vi "Dead Pixel Detection.vi"(0 "image in":refnum<class "MSC Image.lvclass">, 5 "error in (no error)":errorcluster) -> (14 "image out":refnum<class "MSC Image.lvclass">, 15 "mask image out":refnum<class "MSC Image.lvclass">, 19 "error out":errorcluster)   [LabVIEW 2016, in "MSC Image.lvclass"]
doc: "Detects dead pixels through a simple thesholding operation. Use an image with maximum illumination.\n\nYou can use the mask image of the detected pixels with Inpaint to restore the fragments."
uses:
  MSC Image.lvclass
  controls/Image Type.ctl
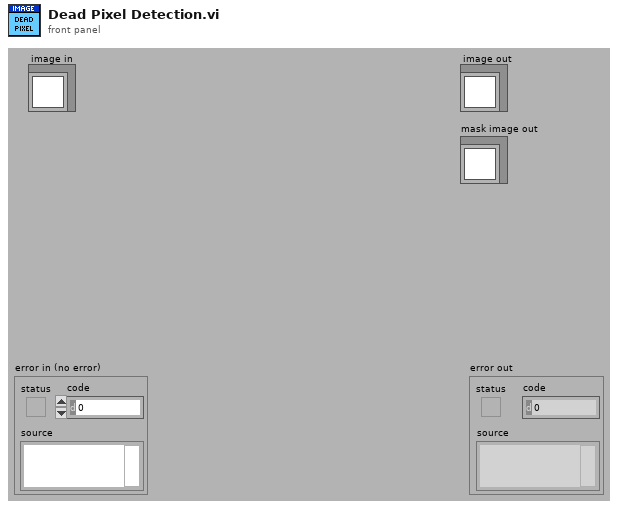
[diagram p1: front panel]
types:
  T1 = typedef "MSC Image.lvclass/Image Type.ctl" = i32
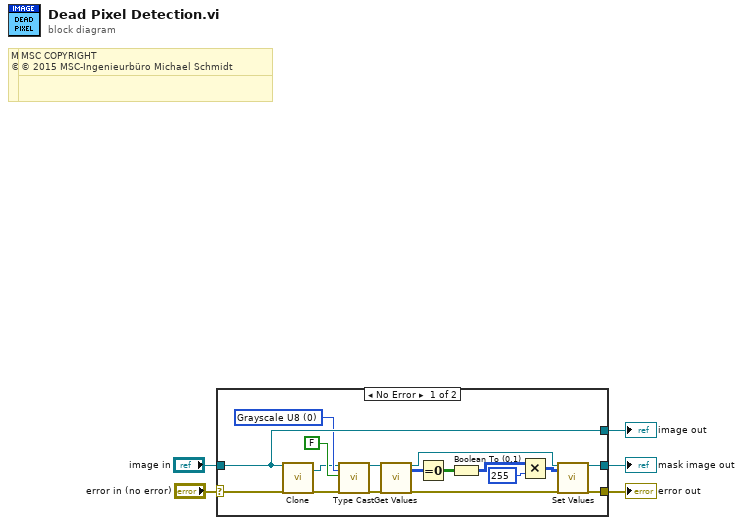
[diagram p0: block diagram]
diagram:
  # "MSC COPYRIGHT\n© 2016 MSC-Ingenieurbüro Michael Schmidt"
  # "MSC COPYRIGHT\n© 2016 MSC-Ingenieurbüro Michael Schmidt"
  # "MSC COPYRIGHT\n© 2015 MSC-Ingenieurbüro Michael Schmidt"
  # "MSC COPYRIGHT\n© 2015 MSC-Ingenieurbüro Michael Schmidt"
  n1 = case shown="No Error" "error in (no error)" {
    selector: "error in (no error)" -> [w8 w24]
    tunnel: [w7 w24] -> w4
    tunnel: [w22 w23] -> w2
    tunnel: "image in" -> [w22 w23]
    tunnel: [w12 _] -> w1
    frame No Error {
      w20 = T1 0 items=["Grayscale U8"=0, "Grayscale U16"=2, "Grayscale Single"=5, "Grayscale Double"=6, "RGB U8"=16] ("Image Type")
      n2 = call-dynamic "Clone.vi"("image in"=w22, "error in (no error)"=w8) -> ("clone image out"=w6:refnum<class "MSC Image.lvclass">, "error out"=w9:errorcluster)  [unwired: 15 in, 1 out]
      n3 = call-dynamic "Type Cast.vi"("image in"=w6, "Image Type"=w20, "Scale?"=FALSE, "error in (no error)"=w9) -> ("image out"=w19:refnum<class "MSC Image.lvclass">, "error out"=w10:errorcluster)  [unwired: 14 in]
      n4 = call-dynamic "Get Values.vi"("image in"=w19, "error in (no error)"=w10) -> ("image out"=w13:refnum<class "MSC Image.lvclass">, "imageData U8"=w15:u8[][], "error out"=w11:errorcluster)  [unwired: 10 in, 5 out]
      n5 = Equal To 0?(x=w15) -> (x = 0?=w16:bool[][])
      n6 = Boolean To (0,1)(Boolean=w16) -> (0, 1=w17:i16[][])
      n7 = Multiply(x=w17, y=255 ("Image Type")) -> (x*y=w14:i32[][])
      n8 = call-dynamic "Set Values.vi"("image in"=w13, "imageData U8"=w14, "error in (no error)"=w11) -> ("image out"=w12:refnum<class "MSC Image.lvclass">, "error out"=w7:errorcluster)  [unwired: 15 in]
    }
    frame Error {
    }
  }
  "error out" <- w4
  "image out" <- w2
  "mask image out" <- w1
